vi "DegtoRads.vi"(11 "Degrees in":dbl) -> (3 "Rads Out":dbl)   [LabVIEW 2011]
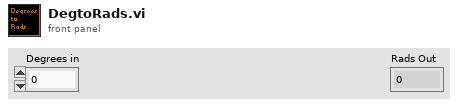
[diagram p1: front panel]
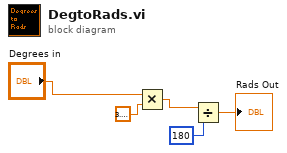
[diagram p0: block diagram]
diagram:
  n1 = Multiply(x="Degrees in", y=3.141592653589793) -> (x*y=w3:dbl)
  n2 = Divide(x=w3, y=180) -> (x/y=→"Rads Out":dbl)
